vi "InstallArduinoLibs.vi"() -> ()   [LabVIEW 2019]
uses:
  <vilib>/Utility/sysdir.llb/System Directory Type.ctl
  vi.lib/LINXx/LINXx.lvlib
panel:
  in  "skip":bool
  in  "copy":bool
  in  "Path":path
  # "Arduino Library Installation"
  # "To complete your installation of LINXx, you need to specify the location of your Arduino sketchbook folder.\nIf you're not sure what that path is, open the Arduino IDE, go to File>Preferences, and copy the path under \"Sketchbook location\"."
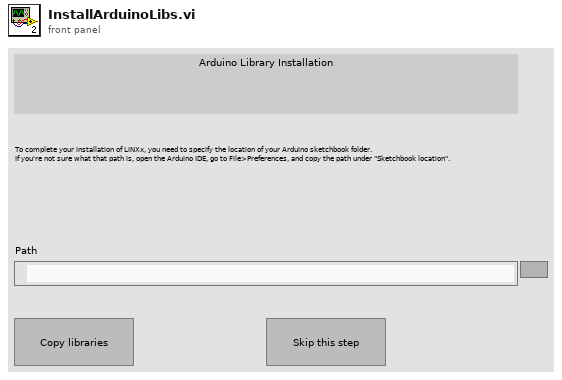
[diagram p1: front panel]
types:
  T1 = typedef "System Directory Type.ctl" = i32
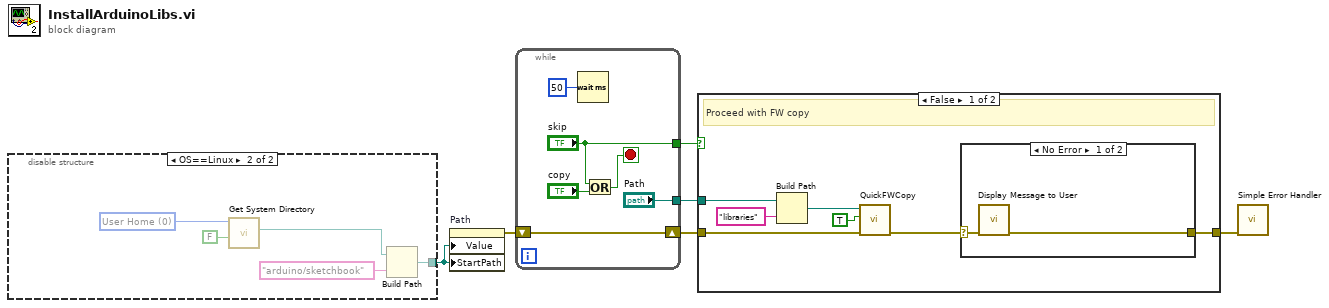
[diagram p0: block diagram]
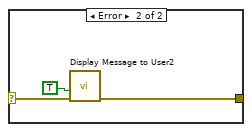
[diagram p2: hidden frame]
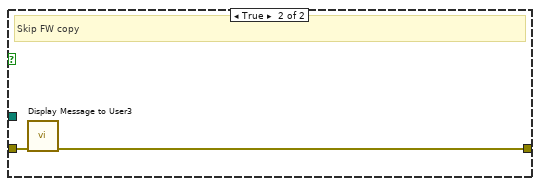
[diagram p3: hidden frame]
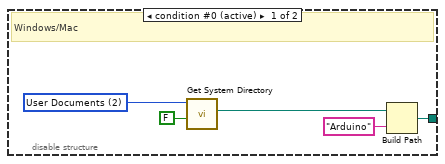
[diagram p4: hidden frame]
diagram:
  n1 = disable-structure shown="OS==Linux" {
    disable-tunnel: [w7 w12] -> w6
    frame condition #0 (active) {
      w8 = T1 2 items=["User Home"=0, "User Desktop"=1, "User Documents"=2, "User Application Data"=3, "User Preferences"=4, "User Temporary"=5, "Public Documents"=6, "Public Application Data"=7, "Public Preferences"=8, "Public Cache"=13, "System Core Libraries"=9, "System Installed Libraries"=10, "Application Files"=11, "Boot Volume Root"=12] ("system directory type")
      # "Windows/Mac"
      n2 = call <vilib>:"Get System Directory.vi"("create directory if not found? (F)"=FALSE, "system directory type"=w8) -> ("system directory"=w11:path)  [unwired: 9 in]
      n3 = Build Path(base path=w11, name or relative path="Arduino") -> (appended path=w7:path)
    }
    frame condition #1 {
      w13 = T1 0 items=["User Home"=0, "User Desktop"=1, "User Documents"=2, "User Application Data"=3, "User Preferences"=4, "User Temporary"=5, "Public Documents"=6, "Public Application Data"=7, "Public Preferences"=8, "Public Cache"=13, "System Core Libraries"=9, "System Installed Libraries"=10, "Application Files"=11, "Boot Volume Root"=12] ("system directory type")
      n4 = call <vilib>:"Get System Directory.vi"("create directory if not found? (F)"=FALSE, "system directory type"=w13) -> ("system directory"=w16:path)  [unwired: 9 in]
      n5 = Build Path(base path=w16, name or relative path="arduino/sketchbook") -> (appended path=w12:path)
    }
  }
  n6 = property on="Path" class="Path"("Value"=w6, "StartPath"=w6) -> (error out=w5:errorcluster)  [unwired: 2 in, 1 out]
  n7 = while {
    tunnel: ["Path"] -> w4
    shift-right: [w20] -> w3
    shift-left: w5 -> [w20]
    tunnel: ["skip"] -> w1
    stop <- w19 stop-if-true
    n8 = Wait (ms)(milliseconds to wait=u32 50) -> ()  [unwired: 1 out]
    n9 = Or(x="skip", y="copy") -> (x .or. y?=w19:bool)
  }
  n10 = case shown="False" w1 {
    tunnel: w4 -> [w29 _]
    tunnel: w3 -> [w27 w36]
    tunnel: [w23 w35] -> w2
    frame False {
      # "Proceed with FW copy"
      n11 = Build Path(base path=w29, name or relative path="libraries") -> (appended path=w25:path)
      n12 = call "QuickFWCopy.vi"("Error In"=w27, "Override lib path?"=TRUE, "Arduino lib directory"=w25) -> ("Error Out"=w24:errorcluster)  [unwired: 8 in]
      n13 = case shown="No Error" w24 {
        selector: w24 -> [w31 w34]
        tunnel: [w30 w33] -> w23
        frame No Error {
          n14 = call "Display Message to User"("error in (no error)"=w31) -> ("error out"=w30:errorcluster)  [unwired: 9 in, 1 out]
        }
        frame Error {
          n15 = call "Display Message to User2"("error in (no error)"=w34, "Enable"=TRUE) -> ("error out"=w33:errorcluster)  [unwired: 8 in, 1 out]
        }
      }
    }
    frame True {
      # "Skip FW copy"
      n16 = call "Display Message to User3"("error in (no error)"=w36) -> ("error out"=w35:errorcluster)  [unwired: 9 in, 1 out]
    }
  }
  n17 = call <vilib>:"Simple Error Handler.vi"("error in (no error)"=w2) -> ()  [unwired: 4 in, 5 out]
